vi "overlay_spot_circle.vi"(5 "error in":errorcluster, 6 "color(black)":u32, 7 "Position":cluster{"x":dbl, "y":dbl, "z":dbl}, 8 "image":T1) -> (0 "error out":errorcluster, 3 "Image Out":T1)   [LabVIEW 2010]
uses:
  <vilib>/vision/Image Controls.llb/IMAQ Image.ctl
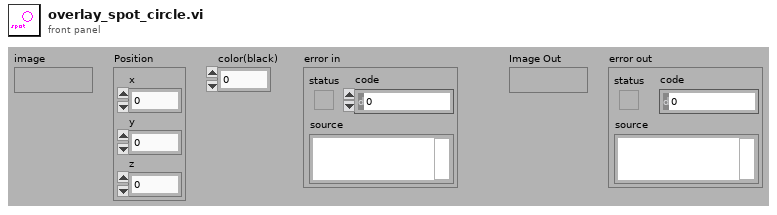
[diagram p1: front panel]
types:
  T1 = typedef "IMAQ Image.ctl" = refnum<image>
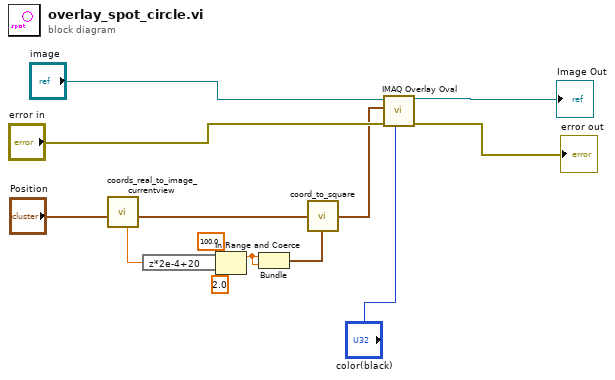
[diagram p0: block diagram]
diagram:
  n1 = call "coords_real_to_image_currentview.vi"("Position (real coords)"="Position") -> ("Position (pixels, relative to the top left of the image)"=w9:cluster{dbl, dbl}, "z (real coords)"=w8:dbl)  [unwired: 7 in]
  n2 = expression code="z*2e-4+20"(w8) -> (w7:dbl)
  n3 = In Range and Coerce(upper limit=100.0, x=w7, lower limit=2.0) -> (coerced(x)=w10:dbl)  [unwired: 1 out]
  n4 = Bundle("upper limit"=w10, "upper limit"=w10) -> (w4:cluster{"upper limit":dbl, "upper limit":dbl})  [unwired: 1 in]
  n5 = call "coord_to_square.vi"("Size"=w4, "Centre"=w9) -> ("rectangle"=w11:cluster{dbl, dbl, dbl, dbl})  [unwired: 2 in]
  n6 = call "IMAQ Overlay Oval"("Color"="color(black)", "error in (no error)"="error in", "Bounding Rectangle"=w11, "Image"="image") -> ("error out"=→"error out":errorcluster, "Image Out"=→"Image Out":T1)  [unwired: 6 in]
